vi "test dummy.vi"(8 "error in (no error)":errorcluster, 11 "Dummy In":refnum<class "Dummy.lvclass">) -> (0 "error out":errorcluster, 3 "Dummy Out":refnum<class "Dummy.lvclass">)   [LabVIEW 2020, in "Dummy.lvclass"]
uses:
  Dummy.lvclass
  Framework/Test Case/LUnit Test Case.lvclass
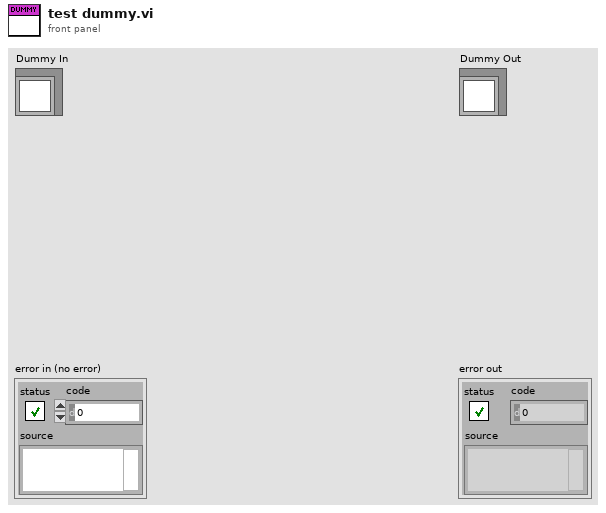
[diagram p1: front panel]
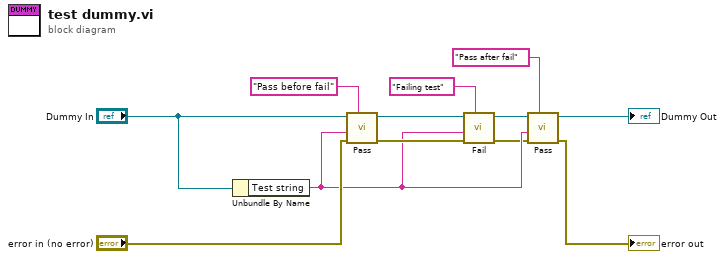
[diagram p0: block diagram]
diagram:
  n1 = Unbundle By Name("Dummy In") -> ("Test string"=w7:string)
  n2 = call "Pass.vi"("Description"="Pass before fail", "error in (no error)"="error in (no error)", "Message"=w7, "LUnit Test Case In"="Dummy In") -> ("error out"=w9:errorcluster, "LUnit Test Case Out"=w10:refnum<class "Dummy.lvclass">)  [unwired: 6 in]
  n3 = call "Fail.vi"("Description"="Failing test", "error in (no error)"=w9, "Message"=w7, "LUnit Test Case In"=w10) -> ("error out"=w4:errorcluster, "LUnit Test Case Out"=w5:refnum<class "Dummy.lvclass">)  [unwired: 6 in]
  n4 = call "Pass.vi"("Description"="Pass after fail", "error in (no error)"=w4, "Message"=w7, "LUnit Test Case In"=w5) -> ("error out"=→"error out":errorcluster, "LUnit Test Case Out"=→"Dummy Out":refnum<class "Dummy.lvclass">)  [unwired: 6 in]
